vi "Inst List Get Labels and Colors.vi"(11 "Instrument List":T2[](array[typedef]) {"Private"."Offset" format="%^_3e"; "Private"."Scale Factors" format="%^_3e"}) -> (0 "Colors":u32[](array[numeric]), 1 "Labels":string[](array[string]), 2 "Number of Columns":u32, 3 "Instrument List Out":T2[](array[typedef]) {"Private"."Offset" format="%^_3e"; "Private"."Scale Factors" format="%^_3e"}, 4 "Display":T1[](array[typedef]), 5 "Scale Factors":dbl[](array[numeric]), 7 "Offsets":dbl[](array[numeric]))   [LabVIEW 2019]
uses:
  Sub Controls/Instrument Properties.ctl
  Sub Controls/Public.ctl
  Sub Controls/Private.ctl
  Sub Controls/Instrument Ref.ctl
  Sub Controls/SystemCheckBox-resize.ctl
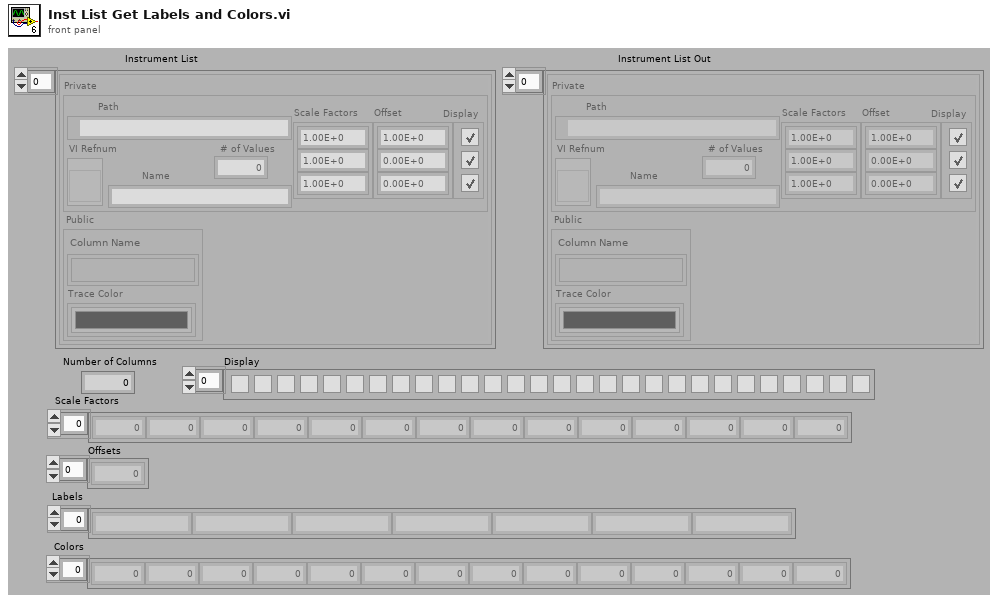
[diagram p1: front panel]
types:
  T1 = typedef "SystemCheckBox-resize.ctl" = bool
  T2 = typedef "Instrument Properties.ctl" = cluster{"Public":T3, "Private":T4}
  T3 = typedef "Public.ctl" = cluster{"Column Name":string[], "Trace Color":u32[]}
  T4 = typedef "Private.ctl" = cluster{"Path":path, "VI Refnum":T5, "Name":string, "# of Values":i32, "Scale Factors":dbl[], "Display":T1[], "Offset":dbl[]}
  T5 = typedef "Instrument Ref.ctl" = refnum<vi>
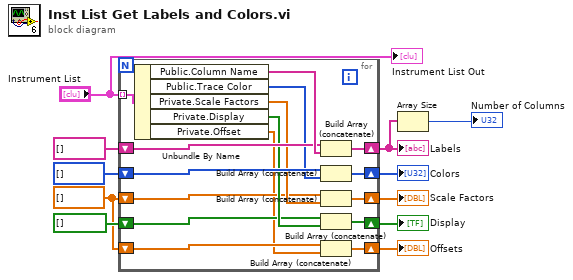
[diagram p0: block diagram]
diagram:
  w2 = dbl[] []
  n1 = for {
    tunnel: "Instrument List" -> [w27] mode=indexing
    shift-right: [w26] -> w7
    shift-left: string[] [] ("Labels") -> [w24]
    shift-right: [w21] -> w8
    shift-left: u32[] [] ("Colors") -> [w23]
    shift-right: [w18] -> w5
    shift-left: w2 -> [w16]
    shift-right: [w19] -> w4
    shift-left: T1[] [] -> [w15]
    shift-right: [w14] -> w1
    shift-left: w2 -> [w13]
    n2 = Unbundle By Name(w27) -> ("Public.Column Name"=w25:string[], "Public.Trace Color"=w22:u32[], "Private.Scale Factors"=w20:dbl[], "Private.Display"=w17:T1[], "Private.Offset"=w12:dbl[])
    n3 = Build Array (concatenate)(w24, w25) -> (w26:string[])
    n4 = Build Array (concatenate)(w23, w22) -> (w21:u32[])
    n5 = Build Array (concatenate)(w16, w20) -> (w18:dbl[])
    n6 = Build Array (concatenate)(w15, w17) -> (w19:T1[])
    n7 = Build Array (concatenate)(w13, w12) -> (w14:dbl[])
  }
  "Colors" <- w8
  "Labels" <- w7
  "Scale Factors" <- w5
  "Display" <- w4
  "Offsets" <- w1
  n8 = Array Size(array=w7) -> (size(s)=→"Number of Columns":i32)
  "Instrument List Out" <- "Instrument List"
